vi "Find Queue By Name.vi"(7 "MsgQ Name":string, 8 "error in (no error)":errorcluster, 11 "Queue references":T1[](array[typedef])) -> (0 "error out":errorcluster, 1 "Queue Index":i32, 2 "Queue Found":bool, 3 "Queue references out":T1[](array[typedef]))   [LabVIEW 2013, in "Interloop MessageQ.lvlib"]
uses:
  Interloop MessageQ.lvlib
  Message Queue Ref.ctl
  Message cluster.ctl
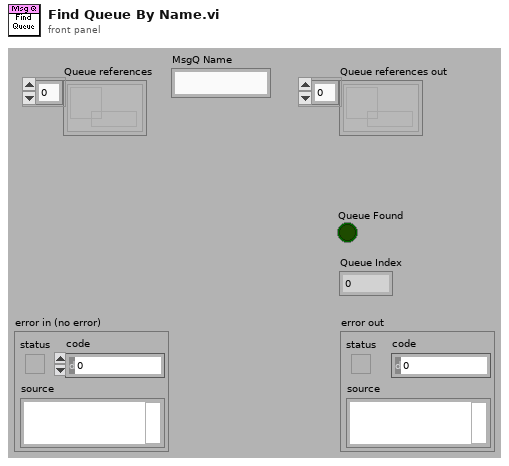
[diagram p1: front panel]
types:
  T1 = typedef "Interloop MessageQ.lvlib/Message Queue Ref.ctl" = refnum<queue>
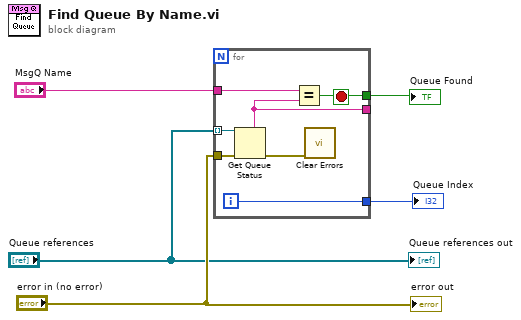
[diagram p0: block diagram]
diagram:
  n1 = for {
    tunnel: "Queue references" -> [w12] mode=indexing
    tunnel: "MsgQ Name" -> [w10]
    tunnel: [w9] -> w4
    tunnel: [w8] -> _
    tunnel: "error in (no error)" -> [w7]
    tunnel: [w6] -> w2
    i -> [w6]
    stop <- w9 stop-if-true
    n2 = Get Queue Status(queue=w12, error in (no error)=w7) -> (queue name=w8:string, error out=w11:errorcluster)  [unwired: 7 out]
    n3 = Equal?(x=w10, y=w8) -> (x = y?=w9:bool)
    n4 = call <vilib>:"Clear Errors.vi"("error in (no error)"=w11) -> ()  [unwired: 7 out]
  }
  "Queue Found" <- w4
  "Queue Index" <- w2
  "error out" <- "error in (no error)"
  "Queue references out" <- "Queue references"
